vi "Active Chal ID FG.vi"(10 "Set?":bool, 11 "Active Chal ID In":i64) -> (3 "Active Chal ID":i64)   [LabVIEW 2020, in "Scores.lvclass"]
uses:
  Scores.lvclass
  Scores.lvclass/Scores.ctl
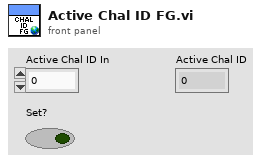
[diagram p1: front panel]
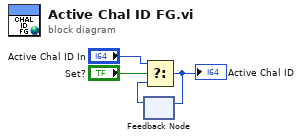
[diagram p0: block diagram]
diagram:
  n1 = feedback #1() -> (w2:i64)  [unwired: 1 in]
  n2 = Select(t="Active Chal ID In", s="Set?", f=w2) -> (s? t:f=w1:i64)
  "Active Chal ID" <- w1
  n3 = feedback-in #1(w1) -> ()
